vi "Set Up 3D Picture.vi"(10 "Reset Camera on Start":bool, 11 "3D Picture Control In":refnum<vi>) -> (2 "Mesh Out":refnum<vi>, 3 "Scene Out":refnum<vi>)   [LabVIEW 2017]
doc: "SubVI for Velodyne HDL-64E S2 Acquire and Graph - 3D.vi. Creates a 3D scene and mesh."
uses:
  <vilib>/Utility/miscctls.llb/LV3DPointTypeDef.ctl
  <vilib>/picture/3D Picture Control/Object/Create Object (name).vi
  <vilib>/picture/3D Picture Control/NI_3D Picture Control.lvlib
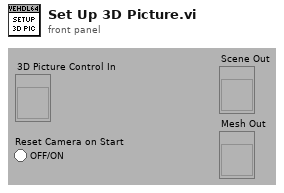
[diagram p1: front panel]
types:
  T1 = typedef "LV3DPointTypeDef.ctl" = cluster{"X":sgl, "Y":sgl, "Z":sgl}
  T2 = enum16{"Inherit Value", "Points", "Wireframe", "Polygons"}
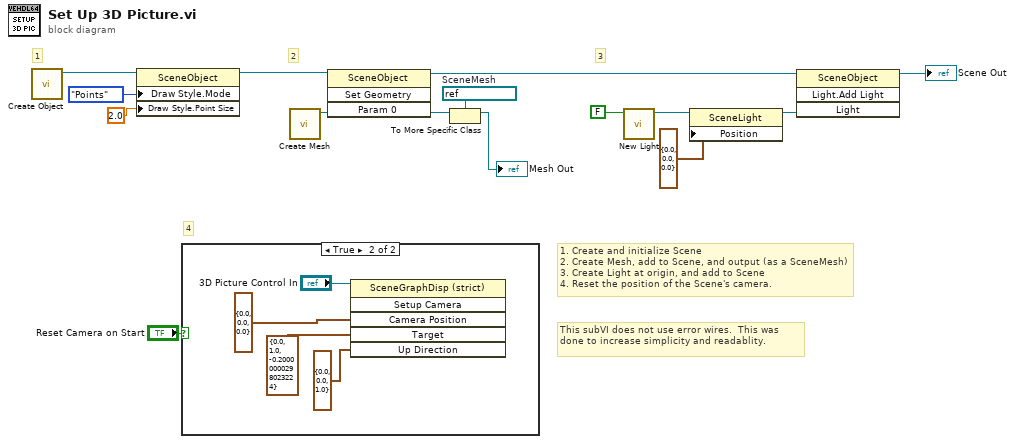
[diagram p0: block diagram]
diagram:
  w8 = refnum<vi> refnum  # SceneMesh
  # "This subVI does not use error wires.  This was done to increase simplicity and readablity."
  # "1. Create and initialize Scene\n2. Create Mesh, add to Scene, and output (as a SceneMesh)\n3. Create Light at origin, and add to Scene\n4. Reset the position of the Scene's camera."
  # "4"
  # "3"
  # "2"
  # "1"
  n1 = call-poly <vilib>:"Create Object.vi"() -> ("Scene:New Object"=w4:refnum<vi>)  [unwired: 10 in, 1 out]
  n2 = property class="SceneObject"(reference=w4, "Draw Style.Mode"=T2."Points" ("Draw Style:Mode"), "Draw Style.Point Size"=sgl 2.0 ("Draw Style:Point Size")) -> (reference out=w10:refnum<vi>)  [unwired: 1 in, 1 out]
  n3 = case shown="True" "Reset Camera on Start" {
    frame False {
    }
    frame True {
      n4 = invoke on="Invoke Node" class="SceneGraphDisp (strict)" method="Setup Camera"(reference="3D Picture Control In", "Camera Position"=T1 {"X"=0.0, "Y"=0.0, "Z"=0.0}, "Target"=T1 {"X"=0.0, "Y"=1.0, "Z"=-0.2}, "Up Direction"=T1 {"X"=0.0, "Y"=0.0, "Z"=1.0}) -> ()  [unwired: 2 in, 6 out]
    }
  }
  n5 = call <vilib>:"Create Mesh.vi"() -> ("New Mesh Refnum"=w7:refnum<vi>)  [unwired: 1 in, 10 out]
  n6 = invoke class="SceneObject" method="Set Geometry"(reference=w10, "Param 0"=w7) -> (reference out=w13:refnum<vi>, "Param 0"=w9:refnum<vi>)  [unwired: 2 in, 2 out]
  n7 = To More Specific Class(target class=w8, reference=w9) -> (specific class reference=→"Mesh Out":refnum<vi>)  [unwired: 1 in, 1 out]
  n8 = call <vilib>:"New Light.vi"("At Infinity"=FALSE) -> ("New Light Refnum"=w11:refnum<vi>)  [unwired: 2 in, 8 out]
  n9 = property class="SceneLight"(reference=w11, "Position"=T1 {"X"=0.0, "Y"=0.0, "Z"=0.0}) -> (reference out=w15:refnum<vi>)  [unwired: 1 in, 1 out]
  n10 = invoke class="SceneObject" method="Light.Add Light"(reference=w13, "Light"=w15) -> (reference out=→"Scene Out":refnum<vi>)  [unwired: 2 in, 3 out]
